vi "AC Output Frequency Test.vi"(7 "Socket":i32, 11 "Scope In":string) -> (0 "error out":errorcluster, 2 "Waveform Data":dbl[](array[numeric]), 3 "Frequency":dbl)   [LabVIEW 2013]
doc: "Measure the frequency of the AC signal. Before calling this VI, ensure that the input signal is set for the battery pin."
uses:
  <vilib>/measure/matone.llb/Extract Single Tone Information 1 Chan.vi
  <instrlib>/Driver Simulation/Oscilloscope.lvlib
  <vilib>/measure/NI_MAPro.lvlib
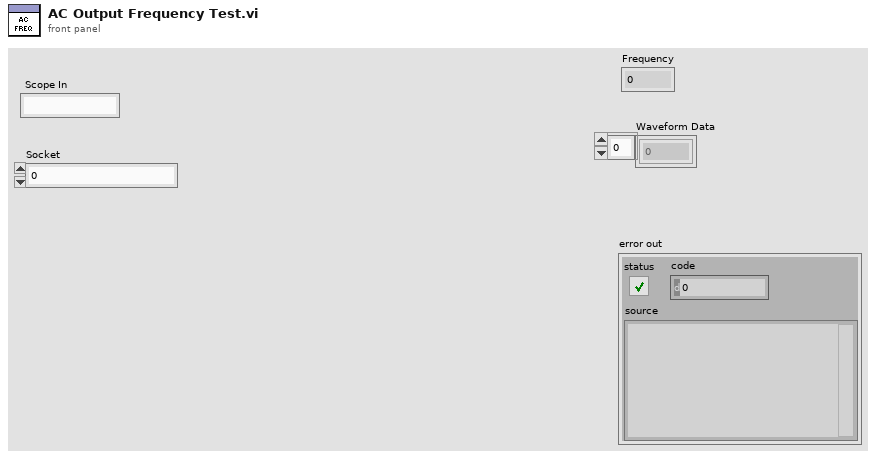
[diagram p1: front panel]
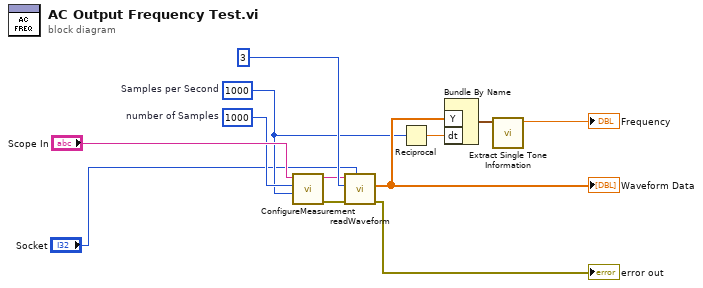
[diagram p0: block diagram]
diagram:
  w3 = 1000  # Samples per Second
  w7 = 1000  # number of Samples
  n1 = call <instrlib>:"ConfigureMeasurement.vi"("Samples Per Second"=w3, "Number of Samples"=w7, "Scope in"="Scope In") -> ("error out"=w9:errorcluster, "Scope out"=w10:string)  [unwired: 7 in]
  n2 = call <instrlib>:"readWaveform.vi"("Test Socket (0)"="Socket", "error in (no error)"=w9, "Channel"=3 ("Scope Channel"), "Scope in"=w10) -> ("error out"=→"error out":errorcluster, "Result"=w4:dbl[])  [unwired: 5 in, 1 out]
  "Waveform Data" <- w4
  n3 = Reciprocal(x=w3) -> (1/x=w6:dbl)
  n4 = Bundle By Name("Y"=w4, "dt"=w6) -> (w5:waveform(dbl))  [unwired: 1 in]
  n5 = call-poly <vilib>:"Extract Single Tone Information.vi"("time signal in"=w5) -> ("detected frequency"=→"Frequency":dbl)  [unwired: 5 in, 5 out]
